vi "Initiate_Handshake.vi"(7 "error in":errorcluster, 10 "Port Number":u16=6123) -> (0 "error out":errorcluster, 2 "WebSocket Connection out":refnum<class "WebSocket Server.lvclass">)   [LabVIEW 2020]
doc: "Reads the TCP Reference number for the given port number"
uses:
  dependencies/WebSockets-API/Source/WebSockets/WebSocket Server/WebSocket Server.lvclass
  dependencies/WebSockets-API/Source/Sockets/VISA TCP Listener/VISA TCP Listener.lvclass
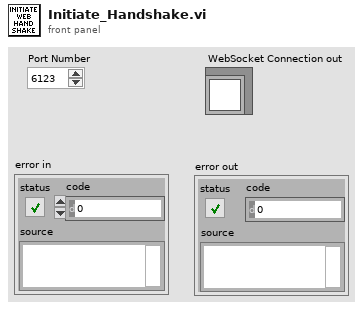
[diagram p1: front panel]
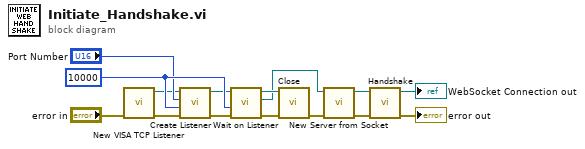
[diagram p0: block diagram]
diagram:
  w15 = 10000 ("timeout ms (25000)")
  n1 = call "New VISA TCP Listener.vi"("error in (no error)"="error in") -> ("error out"=w9:errorcluster, "VISA TCP Listener out"=w8:refnum<class "VISA TCP Listener.lvclass">)  [unwired: 9 in]
  n2 = call-dynamic "Create Listener.vi"("error in (no error)"=w9, "timeout ms (5000)"=w15, "Port"="Port Number", "VISA TCP Listener in"=w8) -> ("error out"=w11:errorcluster, "VISA TCP Listener out"=w13:refnum<class "VISA TCP Listener.lvclass">)  [unwired: 6 in]
  n3 = call-dynamic "Wait on Listener.vi"("error in (no error)"=w11, "timeout ms (5000)"=w15, "VISA TCP Listener in"=w13) -> ("error out"=w10:errorcluster, "Socket out"=w3:refnum<class "Socket.lvclass">, "VISA TCP Listener out"=w12:refnum<class "VISA TCP Listener.lvclass">)  [unwired: 6 in]
  n4 = call-dynamic "Close.vi"("error in (no error)"=w10, "VISA TCP Listener in"=w12) -> ("error out"=w5:errorcluster)  [unwired: 9 in]
  n5 = call "New Server from Socket.vi"("error in (no error)"=w5, "Socket"=w3) -> ("error out"=w6:errorcluster, "WebSocket Server out"=w1:refnum<class "WebSocket Server.lvclass">)  [unwired: 8 in]
  n6 = call-dynamic "Handshake.vi"("error in (no error)"=w6, "WebSocket Connection in"=w1) -> ("error out"=→"error out":errorcluster, "WebSocket Connection out"=→"WebSocket Connection out":refnum<class "WebSocket Server.lvclass">)  [unwired: 8 in]
